vi "UpdateNewTable.vi"(8 "error in (no error)":errorcluster, 10 "index":i32, 11 "List_UI in":refnum<class "List_UI.lvclass">) -> (0 "error out":errorcluster, 3 "List_UI out":refnum<class "List_UI.lvclass">)   [LabVIEW 2015, in "List_UI.lvclass"]
uses:
  List_UI.lvclass
  List_UI.lvclass/List_UI.ctl
  resources/_list/List.lvclass
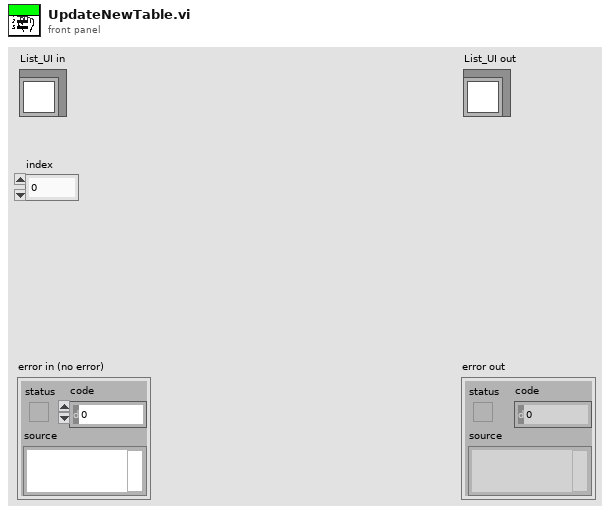
[diagram p1: front panel]
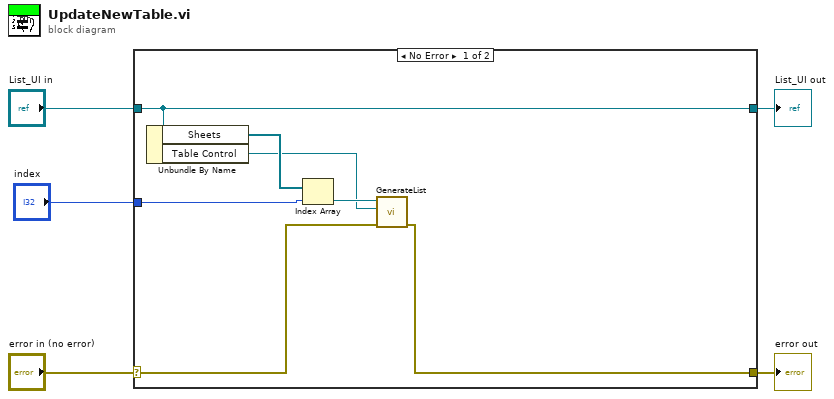
[diagram p0: block diagram]
diagram:
  n1 = case shown="No Error" "error in (no error)" {
    selector: "error in (no error)" -> [w8 w14]
    tunnel: [w6 w14] -> w4
    tunnel: [w12 w13] -> w2
    tunnel: "List_UI in" -> [w12 w13]
    tunnel: "index" -> [w7 _]
    frame No Error {
      n2 = Unbundle By Name(w12) -> ("Sheets"=w11:refnum<class "List.lvclass">[], "Table Control"=w9:refnum<vi>)
      n3 = Index Array(array=w11, index=w7) -> (element=w10:refnum<class "List.lvclass">)
      n4 = call "GenerateList.vi"("error in (no error)"=w8, "reference"=w9, "List in"=w10) -> ("error out"=w6:errorcluster)  [unwired: 7 in, 1 out]
    }
    frame Error {
    }
  }
  "error out" <- w4
  "List_UI out" <- w2
